vi "Introspection Core.vi"(8 "error in (no error)":errorcluster, 11 "BNT_DSCXtGraph in":refnum<class "BNT_DSCXtGraph.lvclass">) -> (0 "error out":errorcluster, 2 "CSPP_Messages":refnum<class "Message.lvclass">[](array[class]), 3 "BNT_DSCXtGraph out":refnum<class "BNT_DSCXtGraph.lvclass">)   [LabVIEW 2017, in "BNT_DSCXtGraph.lvlib" / "BNT_DSCXtGraph.lvclass"]
doc: "This vi delivers a list with all messages this actor reacts to. \n\nNote that all inherited classes have to overwrite it."
uses:
  BNT_DSCXtGraph.lvclass
  <vilib>/ActorFramework/Message/Message.lvclass
  BNT_DSCXtGraph Messages/Read Decimated Traces Msg/Read Decimated Traces Msg.lvclass
  C:/Program Files (x86)/National Instruments/LabVIEW 2017/vi.lib/ActorFramework/Message/Message.lvclass
  BNT_DSCXtGraph Messages/Trace Query Options Msg/Trace Query Options Msg.lvclass
  CSPP_Core/Actors/CSPP_GUIActor/CSPP_GUIActor.lvclass
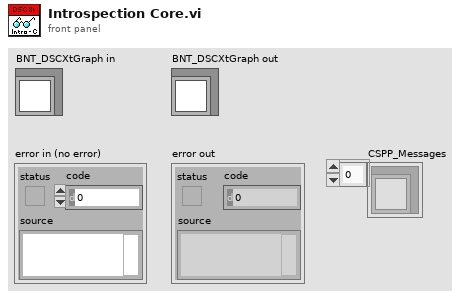
[diagram p1: front panel]
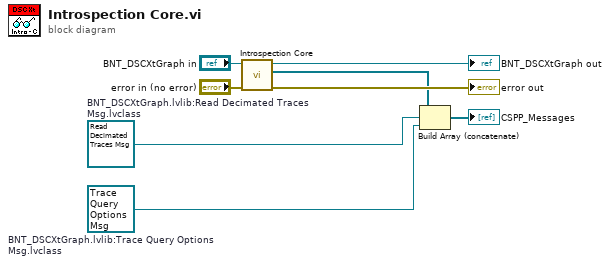
[diagram p0: block diagram]
diagram:
  w1 = refnum<class "Trace Query Options Msg.lvclass"> refnum  # BNT_DSCXtGraph.lvlib:Trace Query Options Msg.lvclass
  w2 = refnum<class "Read Decimated Traces Msg.lvclass"> refnum  # BNT_DSCXtGraph.lvlib:Read Decimated Traces Msg.lvclass
  n1 = call-parent "Introspection Core.vi"("error in (no error)"="error in (no error)", "CSPP_BaseActor in"="BNT_DSCXtGraph in") -> ("error out"=→"error out":errorcluster, "CSPP_Messages"=w7:refnum<class "Message.lvclass">[], "CSPP_BaseActor out"=→"BNT_DSCXtGraph out":refnum<class "BNT_DSCXtGraph.lvclass">)  [unwired: 7 in]
  n2 = Build Array (concatenate)(w7, w2, w1) -> (→"CSPP_Messages":refnum<class "Message.lvclass">[])
